vi "add_txt.vi"() -> ()   [LabVIEW 2016]
uses:
  <vilib>/Utility/file.llb/Read Delimited Spreadsheet (I64).vi
  <vilib>/Utility/file.llb/Write Delimited Spreadsheet (I64).vi
panel:
  out "경로":path
  out "숫자형":i32
  out "추가된 배열":i64[][](array[numeric])
  out "first row":i64[](array[numeric]) caption="첫번째 행"
  in  "Folder Path":path caption="폴더 경로"
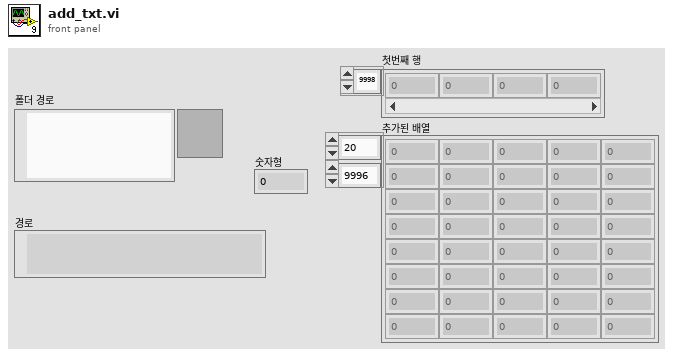
[diagram p1: front panel]
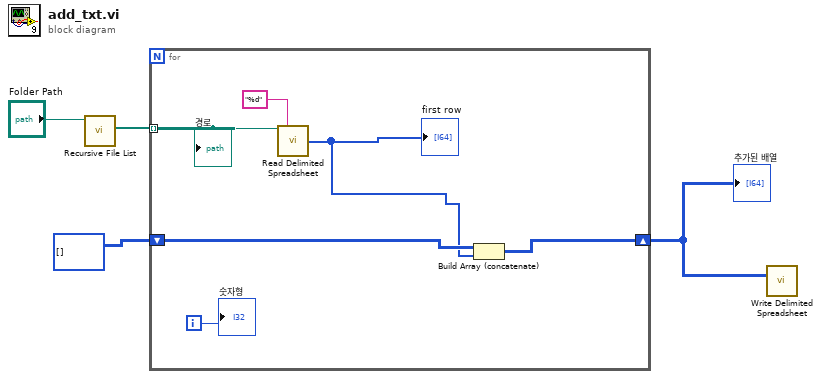
[diagram p0: block diagram]
diagram:
  n1 = call <vilib>:"Recursive File List.vi"("Folder Path"="Folder Path") -> ("All Files in Dir"=w3:path[])  [unwired: 6 in, 4 out]
  n2 = for {
    tunnel: w3 -> [w10] mode=indexing
    shift-right: [w7] -> w1
    shift-left: i64[][] [] ("추가된 배열") -> [w8]
    i -> [w6]
    n3 = call-poly <vilib>:"Read Delimited Spreadsheet.vi"("file path (dialog if empty)"=w10, "format (%d)"="%d") -> ("first row"=w5:i64[])  [unwired: 8 in, 5 out]
    "first row" <- w5
    n4 = Build Array (concatenate)(w8, w5) -> (w7:i64[][])
    "숫자형" <- w6
    "경로" <- w10
  }
  "추가된 배열" <- w1
  n5 = call-poly <vilib>:"Write Delimited Spreadsheet.vi"("2D data"=w1) -> ()  [unwired: 13 in, 2 out]
